vi "IsEvenI16.vi"(4 "x":i16) -> (1 "Even?":bool)   [LabVIEW 2017, in "GPComparison.lvlib"]
doc: "<B>Even?</B> will be True if <B>x</B> is an even integer.\n\nThis VI is inlined.\n\nSteen Schmidt\nGPower\n6/3 2013"
uses:
  GPComparison.lvlib
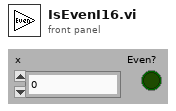
[diagram p1: front panel]
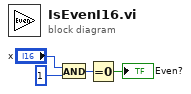
[diagram p0: block diagram]
diagram:
  n1 = And(x="x", y=i16 1) -> (x .and. y?=w4:i16)
  n2 = Equal To 0?(x=w4) -> (x = 0?=→"Even?":bool)
